vi "HCC Get Application Directory.vi"(8 "Error In":errorcluster) -> (0 "Error Out":errorcluster, 1 "General Configuration out":path, 2 "Configuration Path out":path, 3 "Station and Board IDs out":path, 5 "Configuration Path Laundry Lab APP":path, 7 "Software Update Directory":path)   [LabVIEW 2016]
panel:
  out "Application Directory":path
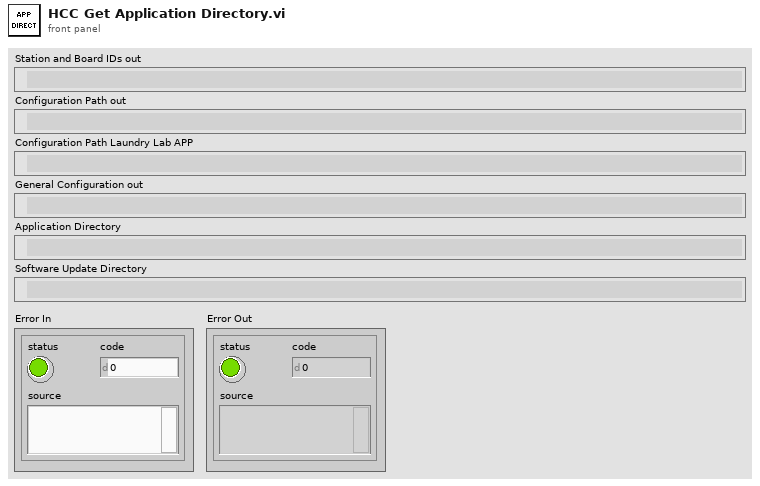
[diagram p1: front panel]
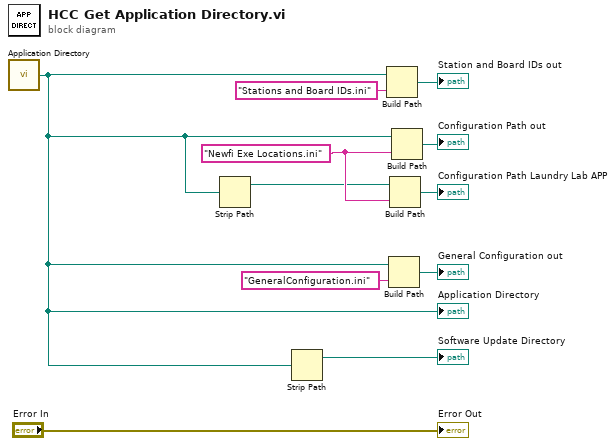
[diagram p0: block diagram]
diagram:
  w5 = "Newfi Exe Locations.ini" ("name or relative path")
  n1 = call <vilib>:"Application Directory.vi"() -> ("Application Directory"=w2:path)
  "Application Directory" <- w2
  n2 = Strip Path(path=w2) -> (stripped path=w4:path)  [unwired: 1 out]
  n3 = Strip Path(path=w2) -> (stripped path=→"Software Update Directory":path)  [unwired: 1 out]
  n4 = Build Path(base path=w2, name or relative path="Stations and Board IDs.ini") -> (appended path=→"Station and Board IDs out":path)
  n5 = Build Path(base path=w2, name or relative path="GeneralConfiguration.ini") -> (appended path=→"General Configuration out":path)
  n6 = Build Path(base path=w4, name or relative path=w5) -> (appended path=→"Configuration Path Laundry Lab APP":path)
  n7 = Build Path(base path=w2, name or relative path=w5) -> (appended path=→"Configuration Path out":path)
  "Error Out" <- "Error In"
